vi "SerialCommunication.Transport.vi"(8 "error in":errorcluster, 9 "Wait For Response?":bool, 10 "Message In":string, 11 "Refnum In":refnum<vi>) -> (0 "error out":errorcluster, 2 "Message Out":string, 3 "Refnum Out":refnum<vi>)   [LabVIEW 2020]
doc: "Use the selected serial comport as the transport method to send and, optionally, receive a message to the target device"
uses:
  <vilib>/Instr/_visa.llb/VISA Configure Serial Port (Instr).vi
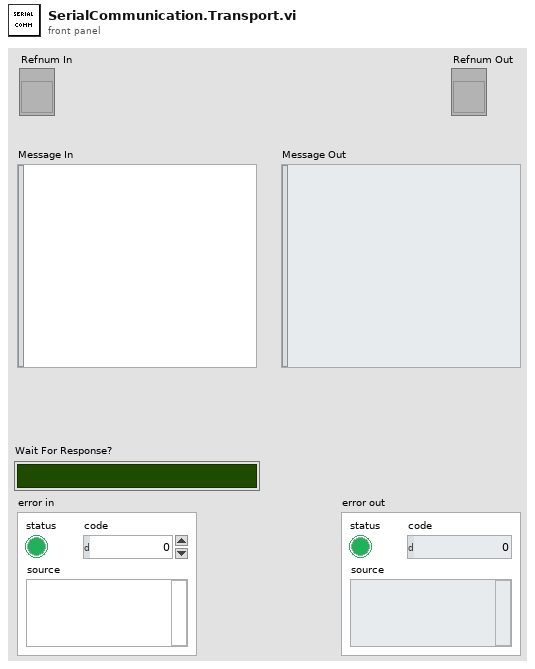
[diagram p1: front panel]
types:
  T1 = typedef "Parameters.ctl" = cluster{"Transport Parameters":T2, "Board Capabilities":map{i32, T4}}
  T2 = typedef "TransportParameters.ctl" = cluster{"Serial Communication":cluster{"Comport":refnum<visa-resource-name>, "No Response Timeout Ms":u32, "Response Complete Timeout Ms":u32, "Max Rx Length":u32, "Baud Rate":u32}, "Selected Transport":T3, "Initializer File Path":path, "Cleaner File Path":path, "Transporter File Path":path}
  T3 = typedef "SupportedTransports.ctl" = enum16{"Serial Communication Port"}
  T4 = typedef "FirmataPinCapabilitiesAndAnalogMapping.ctl" = cluster{"Supported Modes":T5[], "Analog Channel":u8, "Pin Name":string}
  T5 = typedef "FirmataPinCapability.ctl" = cluster{"PinMode":T6, "Resolution":u8}
  T6 = typedef "FirmataPinModes.ctl" = enum16{"DigitalInput", "DigitalOutput", "AnalogInput", "PWM", "Servo", "Shift", "I2C", "OneWire", "Stepper", "Encoder", "Serial", "InputPullup", "Extended.SPI", "Extended.Sonar", "Extended.Tone", "Extended.DHT"}
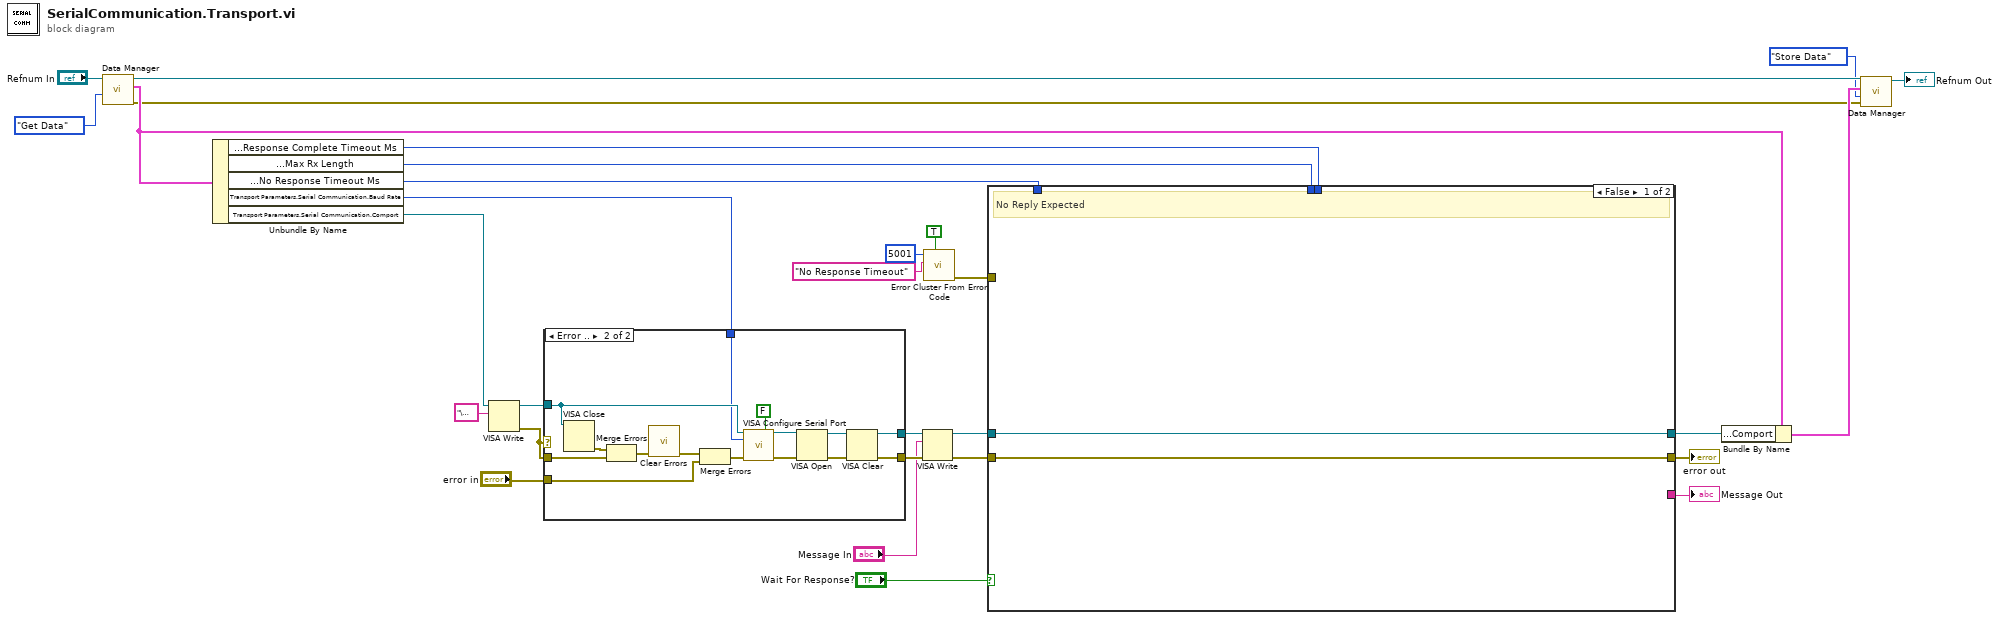
[diagram p0: block diagram]
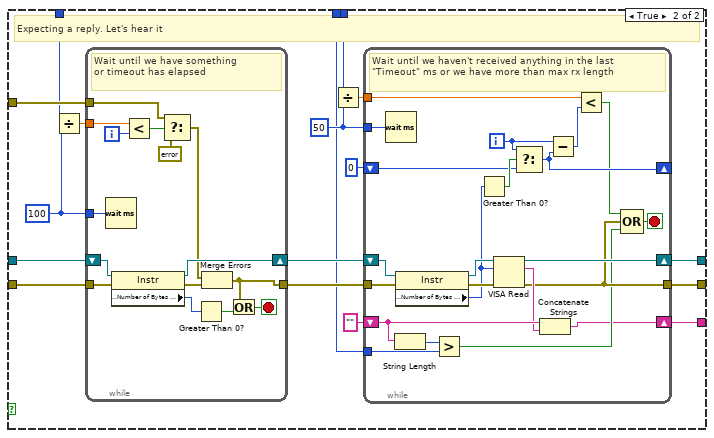
[diagram p2: hidden frame]
diagram:
  n1 = call "Data Manager.vi"("Mode"=enum16{"Store Data", "Get Data", "Cleanup"}."Get Data", "Refnum In"="Refnum In") -> ("error out"=w3:errorcluster, "Data Out"=w9:T1, "Refnum Out"=w6:refnum<vi>)  [unwired: 7 in]
  n2 = Unbundle By Name(w9) -> ("Transport Parameters.Serial Communication.Response Complete Timeout Ms"=w16:u32, "Transport Parameters.Serial Communication.Max Rx Length"=w15:u32, "Transport Parameters.Serial Communication.No Response Timeout Ms"=w17:u32, "Transport Parameters.Serial Communication.Baud Rate"=w13:u32, "Transport Parameters.Serial Communication.Comport"=w14:refnum<visa-resource-name>)
  n3 = VISA Write(VISA resource name=w14, write buffer="\u0000") -> (VISA resource name out=w28:refnum<visa-resource-name>, error out=w26:errorcluster)  [unwired: 1 in, 1 out]
  n4 = case shown="Error .." w26 {
    tunnel: [w32 w37] -> w24
    tunnel: w28 -> [w32 w34]
    tunnel: [w31 w36] -> w25
    tunnel: w26 -> [w31 w43]
    tunnel: "error in" -> [_ w40]
    tunnel: w13 -> [_ w33]
    frame No Error {
    }
    frame Error {
      n5 = VISA Close(VISA resource name=w34) -> (error out=w44:errorcluster)  [unwired: 1 in]
      n6 = Merge Errors(w44, w43) -> (w42:errorcluster)
      n7 = call <vilib>:"Clear Errors.vi"("error in (no error)"=w42) -> ("error out"=w41:errorcluster)  [unwired: 5 in, 1 out]
      n8 = Merge Errors(w41, w40) -> (w47:errorcluster)
      n9 = call-poly "VISA Configure Serial Port"("VISA resource name"=w34, "Enable Termination\nChar (T)"=FALSE ("Enable Termination\nChar (T)"), "baud rate (9600)"=w33, "error in (no error)"=w47) -> ("VISA resource name out"=w45:refnum<visa-resource-name>, "error out"=w46:errorcluster)  [unwired: 10 in]
      n10 = VISA Open(error in (no error)=w46, VISA resource name=w45) -> (VISA resource name=w38:refnum<visa-resource-name>, error out=w39:errorcluster)  [unwired: 3 in]
      n11 = VISA Clear(VISA resource name=w38, error in (no error)=w39) -> (VISA resource name out=w37:refnum<visa-resource-name>, error out=w36:errorcluster)
    }
  }
  n12 = VISA Write(VISA resource name=w24, write buffer="Message In", error in (no error)=w25) -> (VISA resource name out=w23:refnum<visa-resource-name>, error out=w22:errorcluster)  [unwired: 1 out]
  n13 = call <vilib>:"Error Cluster From Error Code.vi"("show call chain? (False)"=TRUE, "error message (\"\")"="No Response Timeout" ("error message (\"\")"), "error code (0)"=5001) -> ("error out"=w18:errorcluster)  [unwired: 6 in]
  n14 = case shown="False" "Wait For Response?" {
    tunnel: w23 -> [w49 w66]
    tunnel: w22 -> [w48 w62]
    tunnel: w18 -> [_ w61]
    tunnel: w17 -> [_ w60]
    tunnel: w16 -> [_ w55]
    tunnel: w15 -> [_ w54]
    tunnel: [_ w52] -> w11
    tunnel: [w48 w51] -> w10
    tunnel: [w49 w50] -> w8
    frame False {
      # "No Reply Expected"
    }
    frame True {
      w59 = u32 50 ("milliseconds to wait")
      w64 = u32 100 ("milliseconds to wait")
      # "Expecting a reply. Let's hear it"
      n15 = Divide(x=w60, y=w64) -> (x/y=w63:dbl)
      n16 = while {
        shift-right: [w102] -> w65
        shift-left: w66 -> [w103]
        tunnel: w64 -> [w100]
        tunnel: w63 -> [w99]
        tunnel: w62 -> [w96]
        tunnel: [w89] -> w56
        tunnel: w61 -> [w93]
        i -> [w98]
        stop <- w97 stop-if-true
        # "Wait until we have something\nor timeout has elapsed"
        n17 = Wait (ms)(milliseconds to wait=w100) -> ()  [unwired: 1 out]
        n18 = property class="Instr"(reference=w103, error in=w96) -> (reference out=w102:refnum<visa-resource-name>, error out=w90:errorcluster, "Serial Settings:Number of Bytes at Serial Port"=w101:u32)
        n19 = Less?(x=w99, y=w98) -> (x < y?=w94:bool)
        n20 = Select(t=w93, s=w94, f=errorcluster {"status"=FALSE, "code"=0, "source"=""}) -> (s? t:f=w91:errorcluster)
        n21 = Greater Than 0?(x=w101) -> (x > 0?=w95:bool)
        n22 = Merge Errors(w91, w90) -> (w89:errorcluster)
        n23 = Or(x=w89, y=w95) -> (x .or. y?=w97:bool)
      }
      n24 = Divide(x=w55, y=w59) -> (x/y=w58:dbl)
      n25 = while {
        shift-right: [w88] -> w50
        shift-left: w65 -> [w85]
        tunnel: w59 -> [w84]
        tunnel: w58 -> [w78]
        shift-right: [w79] -> _
        shift-left: 0 -> [w81]
        tunnel: w56 -> [w76]
        tunnel: [w70] -> w51
        tunnel: w54 -> [w74]
        shift-right: [w67] -> w52
        shift-left: "" -> [w73]
        i -> [w80]
        stop <- w68 stop-if-true
        # "Wait until we haven't received anything in the last \"Timeout\" ms or we have more than max rx length"
        n26 = Wait (ms)(milliseconds to wait=w84) -> ()  [unwired: 1 out]
        n27 = String Length(string=w73) -> (length=w75:i32)
        n28 = property class="Instr"(reference=w85, error in=w76) -> (reference out=w86:refnum<visa-resource-name>, error out=w87:errorcluster, "Serial Settings:Number of Bytes at Serial Port"=w83:u32)
        n29 = Greater?(x=w75, y=w74) -> (0:w69:bool)
        n30 = Greater Than 0?(x=w83) -> (x > 0?=w82:bool)
        n31 = VISA Read(VISA resource name=w86, byte count=w83, error in (no error)=w87) -> (VISA resource name out=w88:refnum<visa-resource-name>, read buffer=w72:string, error out=w70:errorcluster)  [unwired: 1 out]
        n32 = Select(t=w80, s=w82, f=w81) -> (s? t:f=w79:i32)
        n33 = Concatenate Strings(w73, w72) -> (w67:string)
        n34 = Subtract(x=w80, y=w79) -> (x-y=w77:i32)
        n35 = Less?(x=w78, y=w77) -> (x < y?=w71:bool)
        n36 = Compound Arithmetic op=OR(w71, w70, w69) -> (w68:bool)
      }
    }
  }
  "error out" <- w10
  "Message Out" <- w11
  n37 = Bundle By Name(cluster=w9, "Transport Parameters.Serial Communication.Comport"=w8) -> (w4:T1)
  n38 = call "Data Manager.vi"("error in (no error)"=w3, "Mode"=enum16{"Store Data", "Get Data", "Cleanup"}."Store Data", "Data In"=w4, "Refnum In"=w6) -> ("Refnum Out"=→"Refnum Out":refnum<vi>)  [unwired: 5 in, 2 out]
